vi "Keithley2400_LakeShore336_4ProbeResistance_Measurement_DC.vi"() -> ()   [LabVIEW 2018]
uses:
  <instrlib>/Keithley 24XX/Keithley 24XX.lvlib
panel:
  in  "Reset":bool
  in  "Serial Configuration 2":T1={"Baud Rate"=9600, "Parity"=0, "Data Bits"=8, "Stop Bits"=10, "Flow Control"=0} {"Flow Control" items=["None", "XON/XOFF", "RTS/CTS", "XON/XOFF & RTS/CTS", "DTR/DSR", "XON/XOFF & DTR/DSR"]; "Stop Bits" items=["1.0"=10, "1.5"=15, "2.0"=20]; "Data Bits" items=["7"=7, "8"=8]; "Parity" items=["None", "Odd", "Even", "Mark", "Space"]; "Baud Rate" items=["300"=300, "600"=600, "1200"=1200, "2400"=2400, "4800"=4800, "9600"=9600, "19200"=19200]}
  in  "Keithley24XX VISA resource name 2":refnum<visa-resource-name>="GPIB0::21::INSTR" caption="Source Keithley 24XX\nVISA resource name"
  in  "Reset":bool
  in  "Serial Configuration":T1={"Baud Rate"=9600, "Parity"=0, "Data Bits"=8, "Stop Bits"=10, "Flow Control"=0} {"Flow Control" items=["None", "XON/XOFF", "RTS/CTS", "XON/XOFF & RTS/CTS", "DTR/DSR", "XON/XOFF & DTR/DSR"]; "Stop Bits" items=["1.0"=10, "1.5"=15, "2.0"=20]; "Data Bits" items=["7"=7, "8"=8]; "Parity" items=["None", "Odd", "Even", "Mark", "Space"]; "Baud Rate" items=["300"=300, "600"=600, "1200"=1200, "2400"=2400, "4800"=4800, "9600"=9600, "19200"=19200]}
  in  "Keithley24XX VISA resource name":refnum<visa-resource-name>="GPIB0::21::INSTR" caption="Gate Keithley 24XX\nVISA resource name"
  in  "Program Select":enum32{"", "", "", ""}(radio)
  # "(Note, you  may need to set TRUE to get readout working! \nDon't use TRUE when measuring a device!). This program should loop\nthe voltage from the sourcemeter from 0V to 0.5V then jump to 0V and repeat."
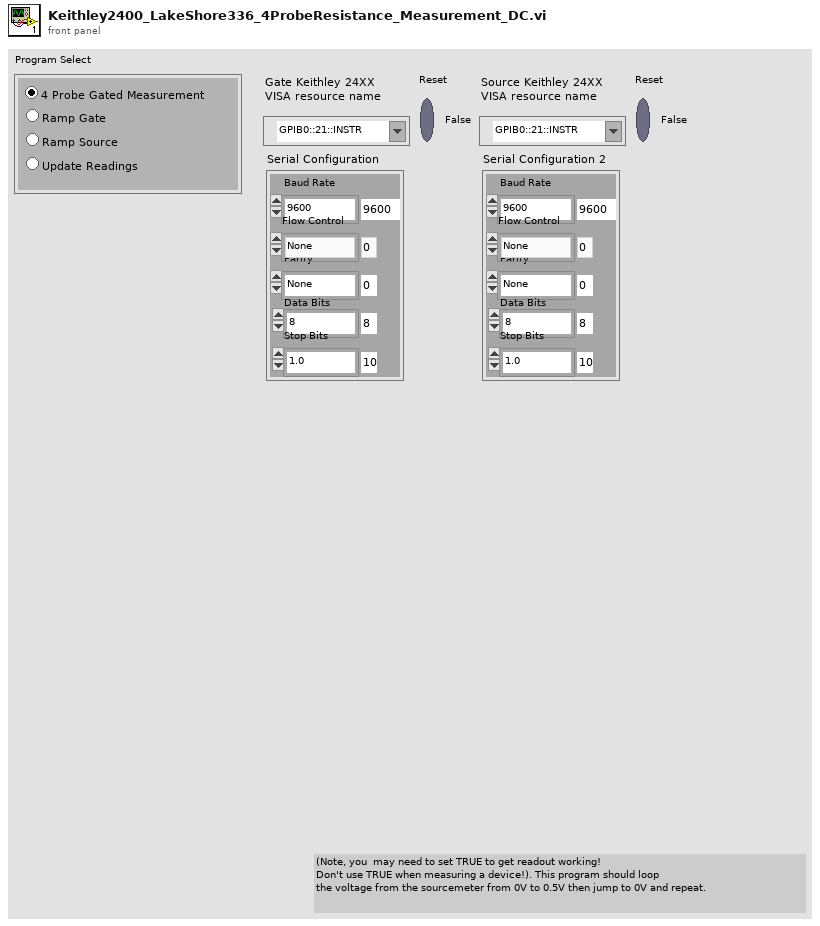
[diagram p1: front panel]
types:
  T1 = cluster{"Baud Rate":u32, "Parity":u16, "Data Bits":u16, "Stop Bits":u16, "Flow Control":u16}
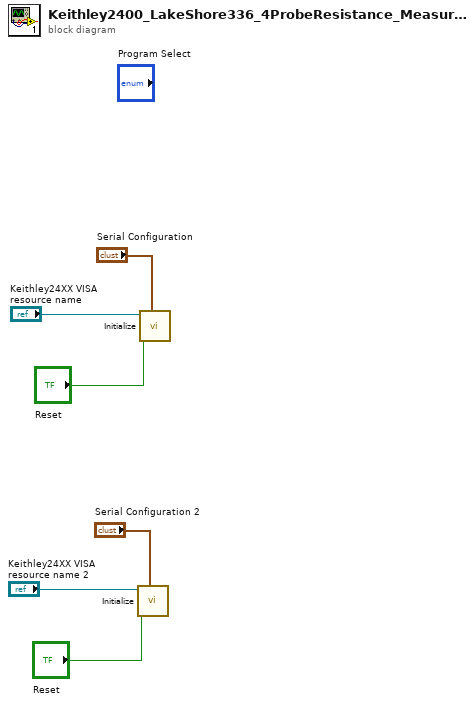
[diagram p0: block diagram]
diagram:
  n1 = call <instrlib>:"Initialize.vi"("Serial Configuration"="Serial Configuration 2", "Reset (True)"="Reset", "VISA resource name"="Keithley24XX VISA resource name 2") -> ()  [unwired: 7 in, 2 out]
  n2 = call <instrlib>:"Initialize.vi"("Serial Configuration"="Serial Configuration", "Reset (True)"="Reset", "VISA resource name"="Keithley24XX VISA resource name") -> ()  [unwired: 7 in, 2 out]
